vi "ReadKeithley6482Configuration.vi"(8 "Error In":errorcluster, 11 "ABLE Config File Ref In":T2) -> (0 "Error Out":errorcluster, 2 "Keithley 6482 Configuration":T1, 3 "ABLE Config File Ref Out":T2)   [LabVIEW 2012]
uses:
  <vilib>/Utility/config.llb/Config Data RefNum.ctl
  Keithley6482Configuration.ctl
  <vilib>/Utility/config.llb/Read Key (String).vi
  <vilib>/Utility/config.llb/NI_LVConfig.lvlib
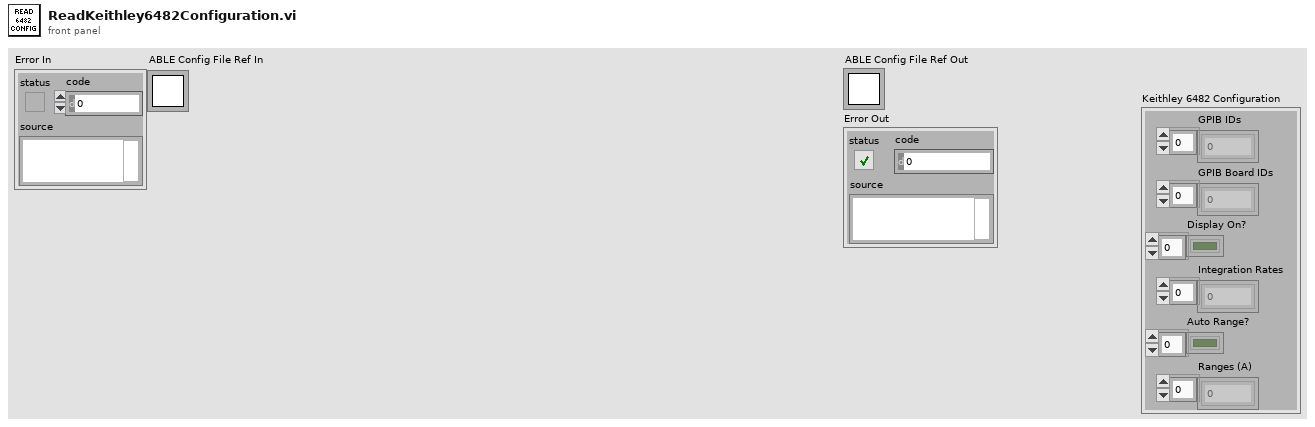
[diagram p1: front panel]
types:
  T1 = typedef "Keithley6482Configuration.ctl" = cluster{"GPIB IDs":u8[], "GPIB Board IDs":u8[], "Display On?":bool[], "Integration Rates":dbl[], "Auto Range?":bool[], "Ranges (A)":dbl[]}
  T2 = typedef "NI_LVConfig.lvlib/Config Data RefNum.ctl" = refnum<k1>
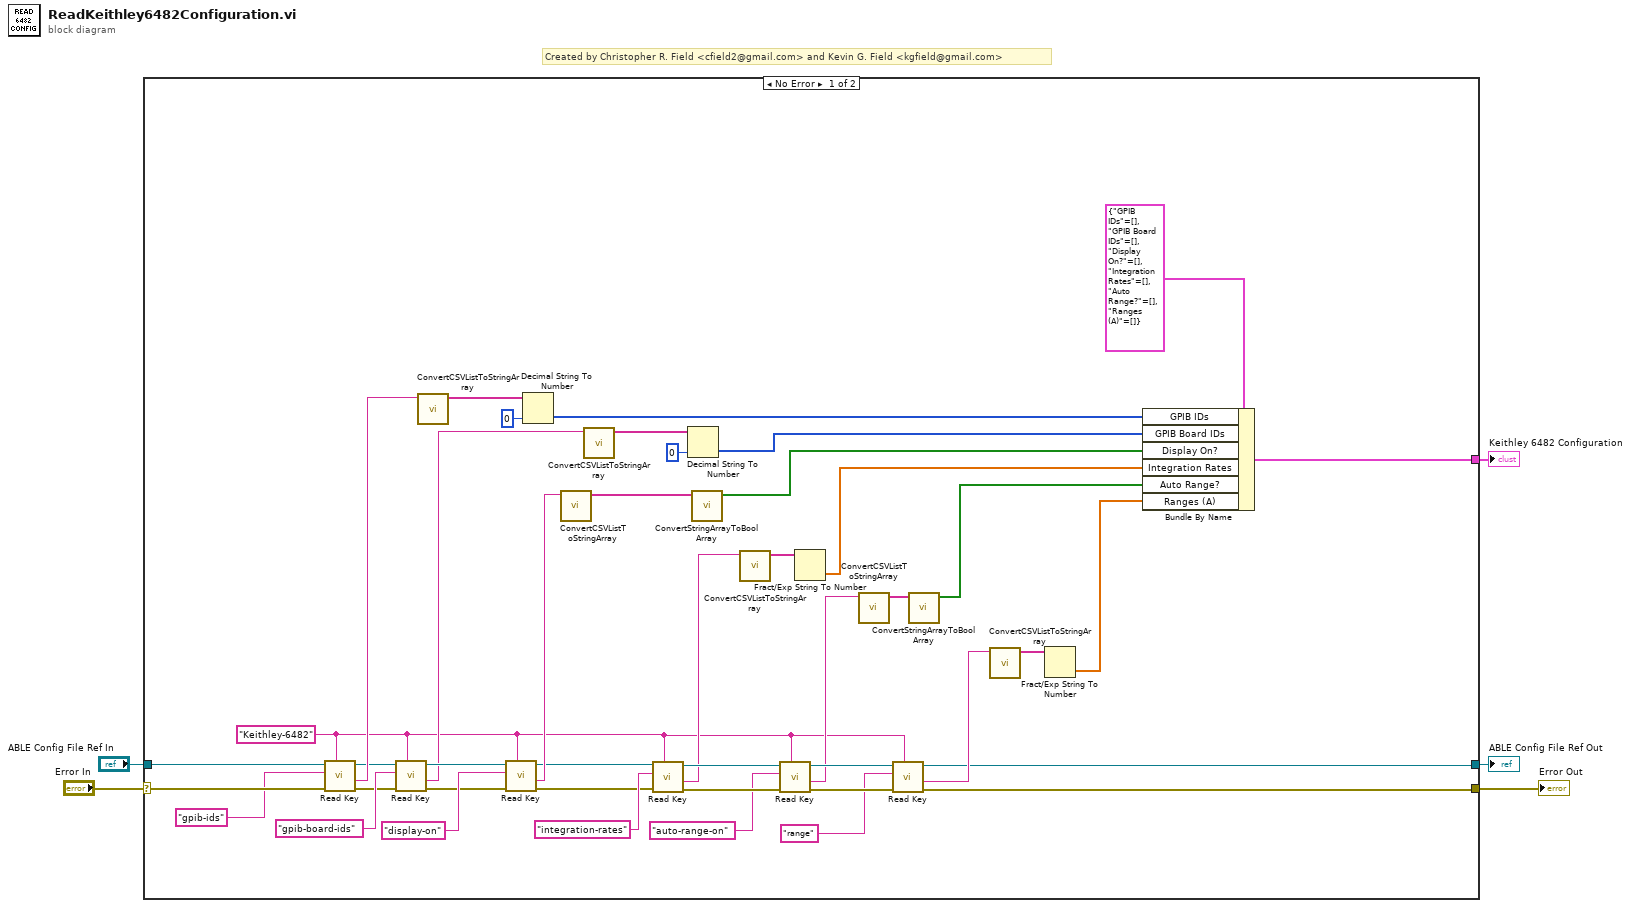
[diagram p0: block diagram]
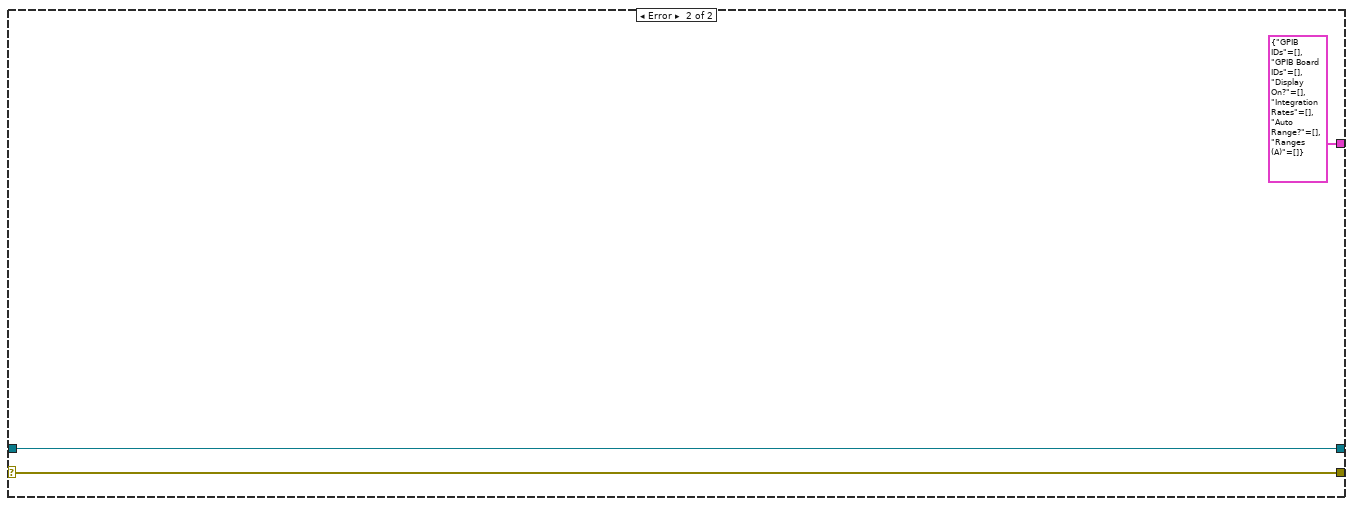
[diagram p2: hidden frame]
diagram:
  # "Created by Christopher R. Field <cfield2@gmail.com> and Kevin G. Field <kgfield@gmail.com>"
  n1 = case shown="No Error" "Error In" {
    selector: "Error In" -> [w48 w50]
    tunnel: "ABLE Config File Ref In" -> [w47 w51]
    tunnel: [w12 w51] -> w3
    tunnel: [w11 w50] -> w2
    tunnel: [w38 T1 {"GPIB IDs"=[], "GPIB Board IDs"=[], "Display On?"=[], "Integration Rates"=[], "Auto Range?"=[], "Ranges (A)"=[]} ("Keithley 6482 Configuration")] -> w1
    frame No Error {
      w13 = "Keithley-6482" ("section")
      n2 = call-poly <vilib>:"Read Key.vi"("section"=w13, "error in (no error)"=w48, "key"="gpib-ids", "refnum"=w47) -> ("error out"=w35:errorcluster, "value"=w44:string, "refnum out"=w36:T2)  [unwired: 4 in, 1 out]
      n3 = call-poly <vilib>:"Read Key.vi"("section"=w13, "error in (no error)"=w35, "key"="gpib-board-ids", "refnum"=w36) -> ("error out"=w34:errorcluster, "value"=w32:string, "refnum out"=w33:T2)  [unwired: 4 in, 1 out]
      n4 = call "ConvertCSVListToStringArray.vi"("CSV List"=w44) -> ("String Array"=w43:string[])  [unwired: 10 in]
      n5 = call-poly <vilib>:"Read Key.vi"("section"=w13, "error in (no error)"=w34, "key"="display-on", "refnum"=w33) -> ("error out"=w14:errorcluster, "value"=w40:string, "refnum out"=w15:T2)  [unwired: 4 in, 1 out]
      n6 = Decimal String To Number(string=w43, default (0L)=u8 0 ("default (0 I32)")) -> (number=w42:u8[])  [unwired: 1 in, 1 out]
      n7 = call "ConvertCSVListToStringArray.vi"("CSV List"=w40) -> ("String Array"=w10:string[])  [unwired: 10 in]
      n8 = call "ConvertCSVListToStringArray.vi"("CSV List"=w32) -> ("String Array"=w31:string[])  [unwired: 10 in]
      n9 = call-poly <vilib>:"Read Key.vi"("section"=w13, "error in (no error)"=w14, "key"="integration-rates", "refnum"=w15) -> ("error out"=w23:errorcluster, "value"=w21:string, "refnum out"=w25:T2)  [unwired: 4 in, 1 out]
      n10 = Decimal String To Number(string=w31, default (0L)=u8 0 ("default (0 I32)")) -> (number=w29:u8[])  [unwired: 1 in, 1 out]
      n11 = call "ConvertStringArrayToBoolArray.vi"("String Array"=w10) -> ("Boolean Array"=w9:bool[])  [unwired: 10 in]
      n12 = call "ConvertCSVListToStringArray.vi"("CSV List"=w21) -> ("String Array"=w28:string[])  [unwired: 10 in]
      n13 = call-poly <vilib>:"Read Key.vi"("section"=w13, "error in (no error)"=w23, "key"="auto-range-on", "refnum"=w25) -> ("error out"=w22:errorcluster, "value"=w19:string, "refnum out"=w24:T2)  [unwired: 4 in, 1 out]
      n14 = Fract/Exp String To Number(string=w28) -> (number=w8:dbl[])  [unwired: 3 in, 1 out]
      n15 = call "ConvertCSVListToStringArray.vi"("CSV List"=w19) -> ("String Array"=w27:string[])  [unwired: 10 in]
      n16 = call-poly <vilib>:"Read Key.vi"("section"=w13, "error in (no error)"=w22, "key"="range", "refnum"=w24) -> ("error out"=w11:errorcluster, "value"=w18:string, "refnum out"=w12:T2)  [unwired: 4 in, 1 out]
      n17 = call "ConvertStringArrayToBoolArray.vi"("String Array"=w27) -> ("Boolean Array"=w7:bool[])  [unwired: 10 in]
      n18 = call "ConvertCSVListToStringArray.vi"("CSV List"=w18) -> ("String Array"=w26:string[])  [unwired: 10 in]
      n19 = Fract/Exp String To Number(string=w26) -> (number=w6:dbl[])  [unwired: 3 in, 1 out]
      n20 = Bundle By Name(cluster=T1 {"GPIB IDs"=[], "GPIB Board IDs"=[], "Display On?"=[], "Integration Rates"=[], "Auto Range?"=[], "Ranges (A)"=[]} ("Keithley 6482 Configuration"), "GPIB IDs"=w42, "GPIB Board IDs"=w29, "Display On?"=w9, "Integration Rates"=w8, "Auto Range?"=w7, "Ranges (A)"=w6) -> (w38:T1)
    }
    frame Error {
    }
  }
  "ABLE Config File Ref Out" <- w3
  "Error Out" <- w2
  "Keithley 6482 Configuration" <- w1
